vi "Scale_Noise_floor_to_dBm.vi"(11 "spectrum in (Volts)":dbl[](array[numeric])) -> (3 "Spectrum_dBm":dbl[](array[numeric]))   [LabVIEW 2018]
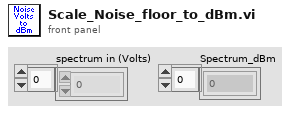
[diagram p1: front panel]
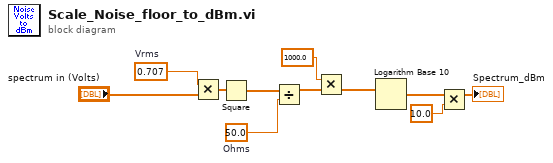
[diagram p0: block diagram]
diagram:
  w3 = 0.707  # Vrms
  w6 = 50.0  # Ohms
  n1 = Multiply(x=w3, y="spectrum in (Volts)") -> (x*y=w1:dbl[])
  n2 = Square(x=w1) -> (x^2=w8:dbl[])
  n3 = Divide(x=w8, y=w6) -> (x/y=w7:dbl[])
  n4 = Multiply(x=1000.0, y=w7) -> (x*y=w5:dbl[])
  n5 = Logarithm Base 10(1:w5) -> (0:w11:dbl[])
  n6 = Multiply(x=w11, y=10.0) -> (x*y=→"Spectrum_dBm":dbl[])
